vi "measurement computing(SubVI).vi"(9 "stop":bool, 10 "TCs 9-16":u16(ring)=1 items=["Dev0", "Dev1", "Dev2", "Dev3", "Dev4", "Dev5", "Dev6", "Dev7"], 11 "TCs 1-8":u16(ring) items=["Dev0", "Dev1", "Dev2", "Dev3", "Dev4", "Dev5", "Dev6", "Dev7"]) -> (3 "data":dbl[](array[numeric]))   [LabVIEW 2012]
uses:
  <vilib>/ULx/Create Channel.llb/ULx Create Channel (AI-Temperature).vi
  <vilib>/ULx/Read.llb/ULx Read (Analog 1D DBL NChan 1Samp).vi
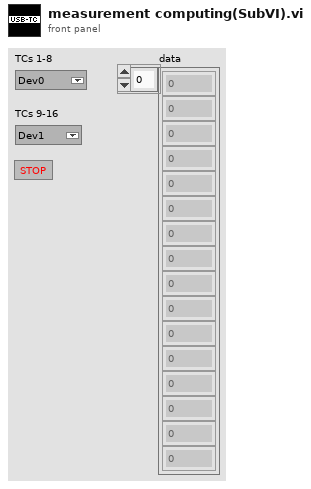
[diagram p1: front panel]
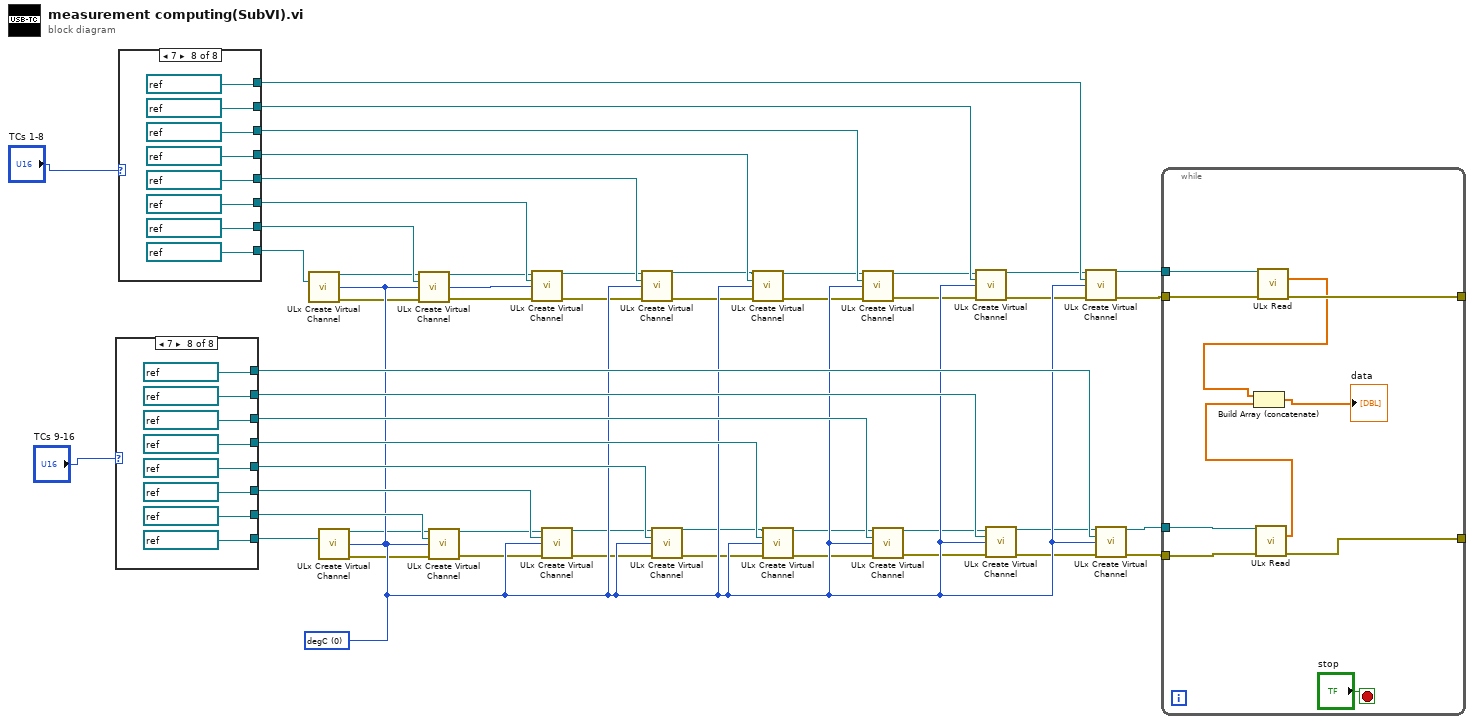
[diagram p0: block diagram]
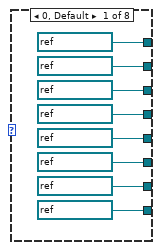
[diagram p2: hidden frame]
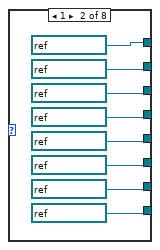
[diagram p3: hidden frame]
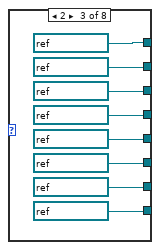
[diagram p4: hidden frame]
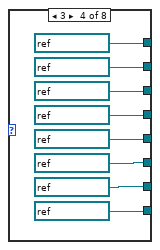
[diagram p5: hidden frame]
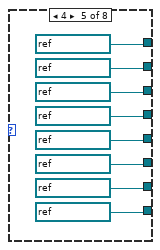
[diagram p6: hidden frame]
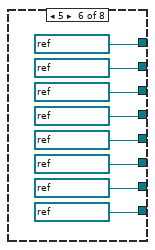
[diagram p7: hidden frame]
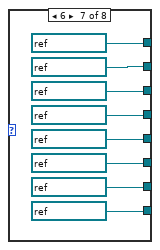
[diagram p8: hidden frame]
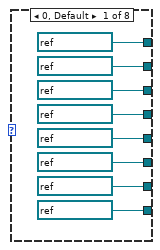
[diagram p9: hidden frame]
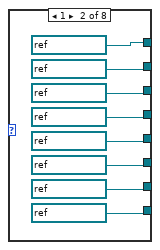
[diagram p10: hidden frame]
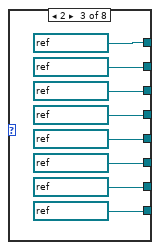
[diagram p11: hidden frame]
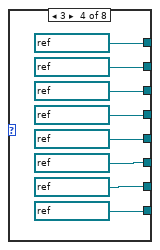
[diagram p12: hidden frame]
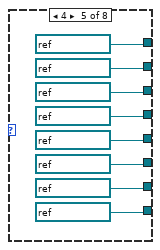
[diagram p13: hidden frame]
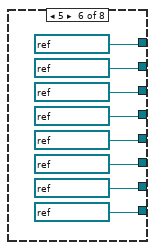
[diagram p14: hidden frame]
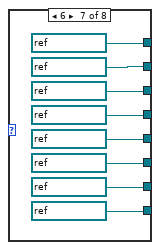
[diagram p15: hidden frame]
diagram:
  w31 = 0 items=["degC", "degF", "kelvin", "raw"] ("units")
  n1 = case shown="7" "TCs 9-16" {
    tunnel: [refnum<k21> "Dev0/Ti7" ("physical channels 2") refnum<k21> "Dev1/Ti7" ("physical channels 2") refnum<k21> "Dev2/Ti7" ("physical channels 2") refnum<k21> "Dev3/Ti7" ("physical channels 2") refnum<k21> "Dev4/Ti7" ("physical channels 2") refnum<k21> "Dev5/Ti7" ("physical channels 2") refnum<k21> "Dev6/Ti7" ("physical channels 2") refnum<k21> "Dev7/Ti7" ("physical channels 2")] -> w47
    tunnel: [refnum<k21> "Dev0/Ti6" ("physical channels") refnum<k21> "Dev1/Ti6" ("physical channels") refnum<k21> "Dev2/Ti6" ("physical channels") refnum<k21> "Dev3/Ti6" ("physical channels") refnum<k21> "Dev4/Ti6" ("physical channels") refnum<k21> "Dev5/Ti6" ("physical channels") refnum<k21> "Dev6/Ti6" ("physical channels") refnum<k21> "Dev7/Ti6" ("physical channels")] -> w46
    tunnel: [refnum<k21> "Dev0/Ti5" ("physical channels 2") refnum<k21> "Dev1/Ti5" ("physical channels 2") refnum<k21> "Dev2/Ti5" ("physical channels 2") refnum<k21> "Dev3/Ti5" ("physical channels 2") refnum<k21> "Dev4/Ti5" ("physical channels 2") refnum<k21> "Dev5/Ti5" ("physical channels 2") refnum<k21> "Dev6/Ti5" ("physical channels 2") refnum<k21> "Dev7/Ti5" ("physical channels 2")] -> w45
    tunnel: [refnum<k21> "Dev0/Ti4" ("physical channels") refnum<k21> "Dev1/Ti4" ("physical channels") refnum<k21> "Dev2/Ti4" ("physical channels") refnum<k21> "Dev3/Ti4" ("physical channels") refnum<k21> "Dev4/Ti4" ("physical channels") refnum<k21> "Dev5/Ti4" ("physical channels") refnum<k21> "Dev6/Ti4" ("physical channels") refnum<k21> "Dev7/Ti4" ("physical channels")] -> w44
    tunnel: [refnum<k21> "Dev0/Ti3" ("physical channels 2") refnum<k21> "Dev1/Ti3" ("physical channels 2") refnum<k21> "Dev2/Ti3" ("physical channels 2") refnum<k21> "Dev3/Ti3" ("physical channels 2") refnum<k21> "Dev4/Ti3" ("physical channels 2") refnum<k21> "Dev5/Ti3" ("physical channels 2") refnum<k21> "Dev6/Ti3" ("physical channels 2") refnum<k21> "Dev7/Ti3" ("physical channels 2")] -> w43
    tunnel: [refnum<k21> "Dev0/Ti2" ("physical channels") refnum<k21> "Dev1/Ti2" ("physical channels") refnum<k21> "Dev2/Ti2" ("physical channels") refnum<k21> "Dev3/Ti2" ("physical channels") refnum<k21> "Dev4/Ti2" ("physical channels") refnum<k21> "Dev5/Ti2" ("physical channels") refnum<k21> "Dev6/Ti2" ("physical channels") refnum<k21> "Dev7/Ti2" ("physical channels")] -> w42
    tunnel: [refnum<k21> "Dev0/Ti1" ("physical channels 2") refnum<k21> "Dev1/Ti1" ("physical channels 2") refnum<k21> "Dev2/Ti1" ("physical channels 2") refnum<k21> "Dev3/Ti1" ("physical channels 2") refnum<k21> "Dev4/Ti1" ("physical channels 2") refnum<k21> "Dev5/Ti1" ("physical channels 2") refnum<k21> "Dev6/Ti1" ("physical channels 2") refnum<k21> "Dev7/Ti1" ("physical channels 2")] -> w41
    tunnel: [refnum<k21> "Dev0/Ti0" ("physical channels") refnum<k21> "Dev1/Ti0" ("physical channels") refnum<k21> "Dev2/Ti0" ("physical channels") refnum<k21> "Dev3/Ti0" ("physical channels") refnum<k21> "Dev4/Ti0" ("physical channels") refnum<k21> "Dev5/Ti0" ("physical channels") refnum<k21> "Dev6/Ti0" ("physical channels") refnum<k21> "Dev7/Ti0" ("physical channels")] -> w40
    frame 0, Default {
    }
    frame 1 {
    }
    frame 2 {
    }
    frame 3 {
    }
    frame 4 {
    }
    frame 5 {
    }
    frame 6 {
    }
    frame 7 {
    }
  }
  n2 = case shown="7" "TCs 1-8" {
    tunnel: [refnum<k21> "Dev0/Ti7" ("physical channels 2") refnum<k21> "Dev1/Ti7" ("physical channels 2") refnum<k21> "Dev2/Ti7" ("physical channels 2") refnum<k21> "Dev3/Ti7" ("physical channels 2") refnum<k21> "Dev4/Ti7" ("physical channels 2") refnum<k21> "Dev5/Ti7" ("physical channels 2") refnum<k21> "Dev6/Ti7" ("physical channels 2") refnum<k21> "Dev7/Ti7" ("physical channels 2")] -> w32
    tunnel: [refnum<k21> "Dev0/Ti6" ("physical channels") refnum<k21> "Dev1/Ti6" ("physical channels") refnum<k21> "Dev2/Ti6" ("physical channels") refnum<k21> "Dev3/Ti6" ("physical channels") refnum<k21> "Dev4/Ti6" ("physical channels") refnum<k21> "Dev5/Ti6" ("physical channels") refnum<k21> "Dev6/Ti6" ("physical channels") refnum<k21> "Dev7/Ti6" ("physical channels")] -> w33
    tunnel: [refnum<k21> "Dev0/Ti5" ("physical channels 2") refnum<k21> "Dev1/Ti5" ("physical channels 2") refnum<k21> "Dev2/Ti5" ("physical channels 2") refnum<k21> "Dev3/Ti5" ("physical channels 2") refnum<k21> "Dev4/Ti5" ("physical channels 2") refnum<k21> "Dev5/Ti5" ("physical channels 2") refnum<k21> "Dev6/Ti5" ("physical channels 2") refnum<k21> "Dev7/Ti5" ("physical channels 2")] -> w34
    tunnel: [refnum<k21> "Dev0/Ti4" ("physical channels") refnum<k21> "Dev1/Ti4" ("physical channels") refnum<k21> "Dev2/Ti4" ("physical channels") refnum<k21> "Dev3/Ti4" ("physical channels") refnum<k21> "Dev4/Ti4" ("physical channels") refnum<k21> "Dev5/Ti4" ("physical channels") refnum<k21> "Dev6/Ti4" ("physical channels") refnum<k21> "Dev7/Ti4" ("physical channels")] -> w35
    tunnel: [refnum<k21> "Dev0/Ti3" ("physical channels 2") refnum<k21> "Dev1/Ti3" ("physical channels 2") refnum<k21> "Dev2/Ti3" ("physical channels 2") refnum<k21> "Dev3/Ti3" ("physical channels 2") refnum<k21> "Dev4/Ti3" ("physical channels 2") refnum<k21> "Dev5/Ti3" ("physical channels 2") refnum<k21> "Dev6/Ti3" ("physical channels 2") refnum<k21> "Dev7/Ti3" ("physical channels 2")] -> w36
    tunnel: [refnum<k21> "Dev0/Ti2" ("physical channels") refnum<k21> "Dev1/Ti2" ("physical channels") refnum<k21> "Dev2/Ti2" ("physical channels") refnum<k21> "Dev3/Ti2" ("physical channels") refnum<k21> "Dev4/Ti2" ("physical channels") refnum<k21> "Dev5/Ti2" ("physical channels") refnum<k21> "Dev6/Ti2" ("physical channels") refnum<k21> "Dev7/Ti2" ("physical channels")] -> w37
    tunnel: [refnum<k21> "Dev0/Ti1" ("physical channels 2") refnum<k21> "Dev1/Ti1" ("physical channels 2") refnum<k21> "Dev2/Ti1" ("physical channels 2") refnum<k21> "Dev3/Ti1" ("physical channels 2") refnum<k21> "Dev4/Ti1" ("physical channels 2") refnum<k21> "Dev5/Ti1" ("physical channels 2") refnum<k21> "Dev6/Ti1" ("physical channels 2") refnum<k21> "Dev7/Ti1" ("physical channels 2")] -> w38
    tunnel: [refnum<k21> "Dev0/Ti0" ("physical channels") refnum<k21> "Dev1/Ti0" ("physical channels") refnum<k21> "Dev2/Ti0" ("physical channels") refnum<k21> "Dev3/Ti0" ("physical channels") refnum<k21> "Dev4/Ti0" ("physical channels") refnum<k21> "Dev5/Ti0" ("physical channels") refnum<k21> "Dev6/Ti0" ("physical channels") refnum<k21> "Dev7/Ti0" ("physical channels")] -> w39
    frame 0, Default {
    }
    frame 1 {
    }
    frame 2 {
    }
    frame 3 {
    }
    frame 4 {
    }
    frame 5 {
    }
    frame 6 {
    }
    frame 7 {
    }
  }
  n3 = call-poly <vilib>:"ULx Create Virtual Channel.vi"("physical channels"=w39, "units"=w31) -> ("task out"=w11:refnum<k24>, "error out"=w12:errorcluster)  [unwired: 12 in]
  n4 = call-poly <vilib>:"ULx Create Virtual Channel.vi"("physical channels"=w40, "units"=w31) -> ("task out"=w22:refnum<k24>, "error out"=w21:errorcluster)  [unwired: 12 in]
  n5 = call-poly <vilib>:"ULx Create Virtual Channel.vi"("task in"=w11, "physical channels"=w38, "units"=w31, "error in"=w12) -> ("task out"=w10:refnum<k24>, "error out"=w9:errorcluster)  [unwired: 10 in]
  n6 = call-poly <vilib>:"ULx Create Virtual Channel.vi"("task in"=w22, "physical channels"=w41, "units"=w31, "error in"=w21) -> ("task out"=w23:refnum<k24>, "error out"=w24:errorcluster)  [unwired: 10 in]
  n7 = call-poly <vilib>:"ULx Create Virtual Channel.vi"("task in"=w10, "physical channels"=w37, "units"=w31, "error in"=w9) -> ("task out"=w14:refnum<k24>, "error out"=w13:errorcluster)  [unwired: 10 in]
  n8 = call-poly <vilib>:"ULx Create Virtual Channel.vi"("task in"=w23, "physical channels"=w42, "units"=w31, "error in"=w24) -> ("task out"=w19:refnum<k24>, "error out"=w20:errorcluster)  [unwired: 10 in]
  n9 = call-poly <vilib>:"ULx Create Virtual Channel.vi"("task in"=w14, "physical channels"=w36, "units"=w31, "error in"=w13) -> ("task out"=w15:refnum<k24>, "error out"=w16:errorcluster)  [unwired: 10 in]
  n10 = call-poly <vilib>:"ULx Create Virtual Channel.vi"("task in"=w19, "physical channels"=w43, "units"=w31, "error in"=w20) -> ("task out"=w18:refnum<k24>, "error out"=w17:errorcluster)  [unwired: 10 in]
  n11 = call-poly <vilib>:"ULx Create Virtual Channel.vi"("task in"=w15, "physical channels"=w35, "units"=w31, "error in"=w16) -> ("task out"=w6:refnum<k24>, "error out"=w5:errorcluster)  [unwired: 10 in]
  n12 = call-poly <vilib>:"ULx Create Virtual Channel.vi"("task in"=w18, "physical channels"=w44, "units"=w31, "error in"=w17) -> ("task out"=w27:refnum<k24>, "error out"=w28:errorcluster)  [unwired: 10 in]
  n13 = call-poly <vilib>:"ULx Create Virtual Channel.vi"("task in"=w6, "physical channels"=w34, "units"=w31, "error in"=w5) -> ("task out"=w7:refnum<k24>, "error out"=w8:errorcluster)  [unwired: 10 in]
  n14 = call-poly <vilib>:"ULx Create Virtual Channel.vi"("task in"=w27, "physical channels"=w45, "units"=w31, "error in"=w28) -> ("task out"=w26:refnum<k24>, "error out"=w25:errorcluster)  [unwired: 10 in]
  n15 = call-poly <vilib>:"ULx Create Virtual Channel.vi"("task in"=w7, "physical channels"=w33, "units"=w31, "error in"=w8) -> ("task out"=w3:refnum<k24>, "error out"=w4:errorcluster)  [unwired: 10 in]
  n16 = call-poly <vilib>:"ULx Create Virtual Channel.vi"("task in"=w26, "physical channels"=w46, "units"=w31, "error in"=w25) -> ("task out"=w30:refnum<k24>, "error out"=w29:errorcluster)  [unwired: 10 in]
  n17 = call-poly <vilib>:"ULx Create Virtual Channel.vi"("task in"=w3, "physical channels"=w32, "units"=w31, "error in"=w4) -> ("task out"=w1:refnum<k24>, "error out"=w2:errorcluster)  [unwired: 10 in]
  n18 = call-poly <vilib>:"ULx Create Virtual Channel.vi"("task in"=w30, "physical channels"=w47, "units"=w31, "error in"=w29) -> ("task out"=w48:refnum<k24>, "error out"=w49:errorcluster)  [unwired: 10 in]
  n19 = while {
    tunnel: w1 -> [w188]
    tunnel: w2 -> [w187]
    tunnel: [w186] -> _
    tunnel: [w185] -> _
    tunnel: w48 -> [w184]
    tunnel: w49 -> [w183]
    stop <- "stop" stop-if-true
    n20 = call-poly <vilib>:"ULx Read.vi"("task in"=w184, "error in"=w183) -> ("data"=w181:dbl[], "error out"=w185:errorcluster)  [unwired: 11 in, 1 out]
    n21 = call-poly <vilib>:"ULx Read.vi"("task in"=w188, "error in"=w187) -> ("data"=w182:dbl[], "error out"=w186:errorcluster)  [unwired: 11 in, 1 out]
    n22 = Build Array (concatenate)(w182, w181) -> (→"data":dbl[])
  }
